vi "max_resource_array_size.vi"(9 "max rows":u32=8, 10 "Resources in":refnum<k20>[](array[refnum])) -> (1 "size > max rows":bool, 2 "array size":u32)   [LabVIEW 2015]
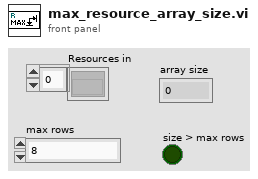
[diagram p1: front panel]
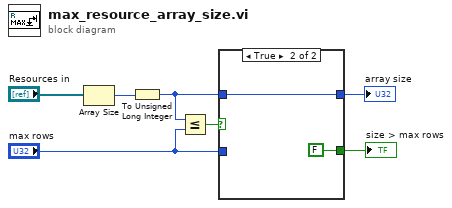
[diagram p0: block diagram]
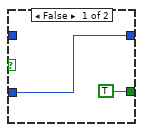
[diagram p2: hidden frame]
diagram:
  n1 = Array Size(array="Resources in") -> (size(s)=w7:i32)
  n2 = To Unsigned Long Integer(number=w7) -> (unsigned 32bit integer=w5:u32)
  n3 = Less Or Equal?(x=w5, y="max rows") -> (x <= y?=w6:bool)
  n4 = case shown="True" w6 {
    tunnel: w5 -> [_ w11]
    tunnel: [w8 w11] -> w4
    tunnel: [TRUE FALSE] -> w3
    tunnel: "max rows" -> [w8 _]
    frame False {
    }
    frame True {
    }
  }
  "array size" <- w4
  "size > max rows" <- w3
